vi "Set verify setting.vi"(0 "VISA Refnum in":refnum<visa-resource-name>, 5 "Set Cmd":string="9999", 7 "Verify cmd":string, 9 "Verify response":string, 11 "error in (no error)":errorcluster) -> (4 "VISA Refnum out":refnum<visa-resource-name>, 6 "Response valid?":bool, 8 "Response":string, 15 "error out":errorcluster)   [LabVIEW 2013]
uses:
  Skywire cmds.ctl
  Test Support VI/String compare type.ctl
panel:
  out "Wait for response msecs":dbl
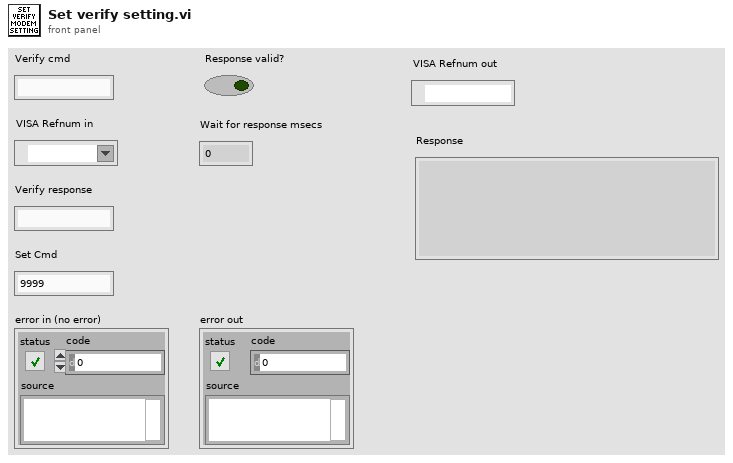
[diagram p1: front panel]
types:
  T1 = typedef "String compare type.ctl" = enum16{"String is exactly response", "String in response somewhere", "String not in response"}
  T2 = typedef "Skywire cmds.ctl" = enum16{"Get primary RSSI", "Get firmware version", "Check 2/3G network reception", "Check LTE network reception", "Get MEID for CDMA", "Get IMEI for 4G/LTE", "Get GPS Coordinates", "Send cmd string", "Check communications", "Enable sim detect", "Check diversity RSSI", "Get make model", "Sierra enable sim det", "get ccid sim id", "Get Gemalto Net Reg", "Get Gemalto model", "Get modem serial number", "Telit sim detect"}
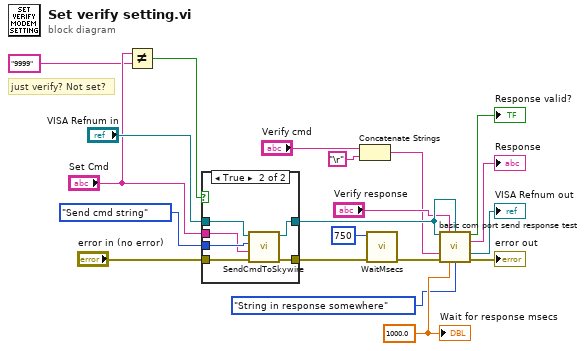
[diagram p0: block diagram]
diagram:
  w19 = 1000.0 ("Wait for response msecs")
  # "just verify? Not set?"
  n1 = Not Equal?(x="Set Cmd", y="9999") -> (x != y?=w1:bool)
  n2 = case shown="True" w1 {
    tunnel: Skywire_cmds."Send cmd string" ("Cmd") -> [_ w28]
    tunnel: "error in (no error)" -> [w22 w27]
    tunnel: [w22 w26] -> w12
    tunnel: [w21 w25] -> w11
    tunnel: "Set Cmd" -> [_ w24]
    tunnel: "VISA Refnum in" -> [w21 w23]
    frame False {
    }
    frame True {
      n3 = call "SendCmdToSkywire.vi"("error in (no error)"=w27, "Cmd String"=w24, "Cmd"=w28, "VISA resource name"=w23) -> ("error out"=w26:errorcluster, "VISA resource name 2"=w25:refnum<visa-resource-name>)  [unwired: 1 in, 5 out]
    }
  }
  n4 = Concatenate Strings("Verify cmd", "\r") -> (w6:string)
  n5 = call "WaitMsecs.vi"("error in (no error)"=w12, "Wait Msecs"=u32 750) -> ("error out"=w13:errorcluster)  [unwired: 9 in]
  n6 = call "basic com port send response test.vi"("VISA Send port"=w11, "Expected response"="Verify response", "VISA Response Port"=w11, "Send text"=w6, "error in (no error)"=w13, "Wait for response msecs"=w19, "Comparison type"=String_compare_type."String in response somewhere") -> ("Response valid?"=→"Response valid?":bool, "Response"=→"Response":string, "VISA Response Port out"=→"VISA Refnum out":refnum<visa-resource-name>, "error out"=→"error out":errorcluster)  [unwired: 4 in, 1 out]
  "Wait for response msecs" <- w19
